vi "Read DMM.vi"(8 "error in (no error)":errorcluster, 11 "DMM Driver in":refnum<class "DMM Driver.lvclass">) -> (0 "error out":errorcluster, 3 "DMM Driver out":refnum<class "DMM Driver.lvclass">)   [LabVIEW 2020, in "DMM Driver.lvclass"]
uses:
  DMM Driver.lvclass
  DMM Driver.lvclass/DMM Driver.ctl
  DMM/DMM.lvclass/DMM.ctl
  DMM/DMM.lvclass
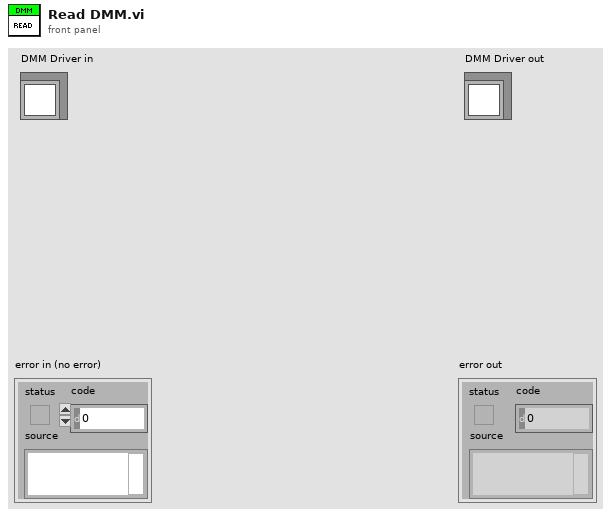
[diagram p1: front panel]
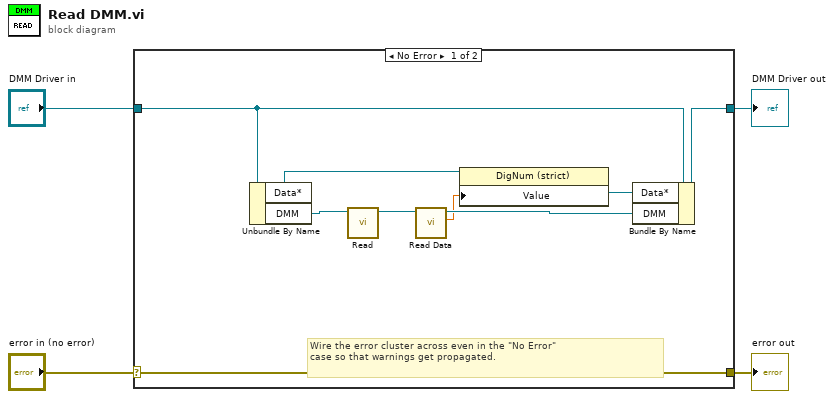
[diagram p0: block diagram]
diagram:
  n1 = case shown="No Error" "error in (no error)" {
    selector: "error in (no error)" -> [w13 w15]
    tunnel: [w13 w15] -> w3
    tunnel: [w10 w14] -> w1
    tunnel: "DMM Driver in" -> [w11 w14]
    frame No Error {
      # "Wire the error cluster across even in the \"No Error\"\ncase so that warnings get propagated."
      n2 = Unbundle By Name(w11) -> ("Data*"=w7:refnum<vi>, "DMM"=w12:refnum<class "DMM.lvclass">)
      n3 = call-dynamic "Read.vi"("DMM in"=w12) -> ("DMM out"=w9:refnum<class "DMM.lvclass">)  [unwired: 9 in, 1 out]
      n4 = call "Read Data.vi"("DMM in"=w9) -> ("Data"=w6:dbl, "DMM out"=w8:refnum<class "DMM.lvclass">)  [unwired: 8 in, 1 out]
      n5 = property class="DigNum (strict)"(reference=w7, "Value"=w6) -> (reference out=w5:refnum<vi>)  [unwired: 1 in, 1 out]
      n6 = Bundle By Name(cluster=w11, "Data*"=w5, "DMM"=w8) -> (w10:refnum<class "DMM Driver.lvclass">)
    }
    frame Error {
    }
  }
  "error out" <- w3
  "DMM Driver out" <- w1
